vi "Write Transfers.vi"(8 "error in (no error)":errorcluster, 10 "Transfers":refnum<class "Configuration.Transfer.lvclass">[](array[class]), 11 "Configuration.Transfer Group in":refnum<class "Configuration.Transfer Group.lvclass">) -> (0 "error out":errorcluster, 3 "Configuration.Transfer Group out":refnum<class "Configuration.Transfer Group.lvclass">)   [LabVIEW 2016, in "Configuration.Transfer Group.lvclass"]
uses:
  Configuration.Transfer Group.lvclass
  Configuration.Transfer/Configuration.Transfer.lvclass
  Configuration.Transfer Group.lvclass/Configuration.Transfer Group.ctl
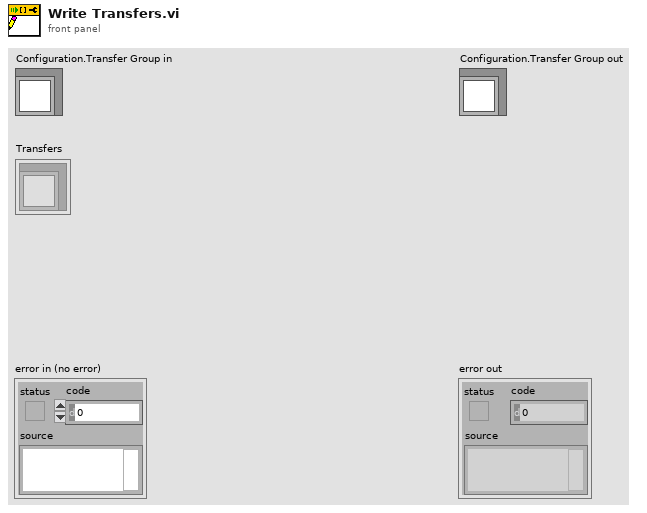
[diagram p1: front panel]
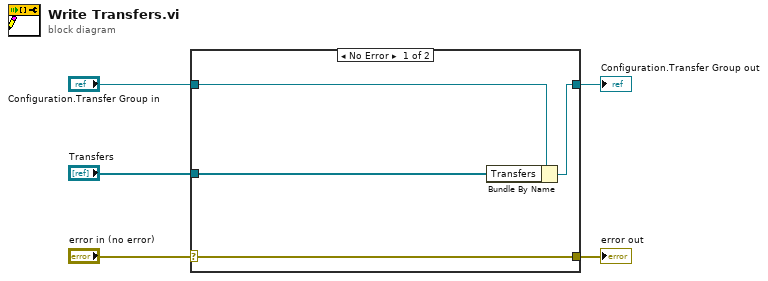
[diagram p0: block diagram]
diagram:
  n1 = case shown="No Error" "error in (no error)" {
    selector: "error in (no error)" -> [w9 w10]
    tunnel: [w9 w10] -> w4
    tunnel: [w7 w11] -> w2
    tunnel: "Configuration.Transfer Group in" -> [w8 w11]
    tunnel: "Transfers" -> [w6 _]
    frame No Error {
      n2 = Bundle By Name(cluster=w8, "Transfers"=w6) -> (w7:refnum<class "Configuration.Transfer Group.lvclass">)
    }
    frame Error {
    }
  }
  "error out" <- w4
  "Configuration.Transfer Group out" <- w2
